vi "Real Matrix Condition Number.vi"(2 "norm type":T1 items=["2-norm", "1-norm", "F-norm", "Inf-norm"], 3 "Input Matrix":T2) -> (0 "error":i32, 1 "condition number":dbl format="%.4f")   [LabVIEW 2020, in "NI_AALPro.lvlib"]
doc: "Computes the <B>condition number</B> of <B>Input Matrix</B>. Wire data to the <B>Input Matrix</B> input to determine the polymorphic instance to use or manually select the instance."
uses:
  NI_AALPro.lvlib
  RealMatrix.ctl
  Matrix Norm Type.ctl
  <resource>/lvanlys.dll
  NI_Matrix.lvlib
panel:
  # "Matrix Condition Number"
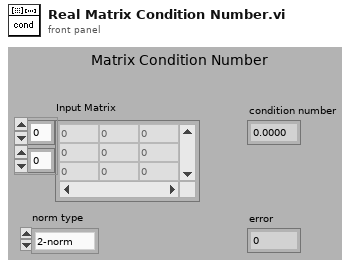
[diagram p1: front panel]
types:
  T1 = typedef "NI_AALPro.lvlib/Matrix Norm Type.ctl" = i32
  T2 = typedef "NI_Matrix.lvlib/RealMatrix.ctl" = dbl[][]
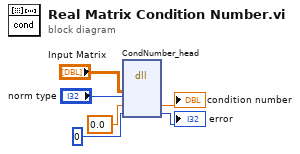
[diagram p0: block diagram]
diagram:
  n1 = dll-call lib="C:/Program Files (x86)/National Instruments/LabVIEW 2020/resource/lvanlys.*" fn="CondNumber_head"("Input Matrix"="Input Matrix", "norm type"="norm type", "condition number"=0.0, "error"=0) -> ("condition number"=→"condition number":dbl, "error"=→"error":i32)  [unwired: 6 in, 2 out]
